vi "INST_PS_SET_CURRENT_LEVEL_4.0.0.vi"(4 "Use OPC(T)":bool, 6 "Instrument Select (Output 1)":string(combo), 7 "SEL_PS":string(combo), 8 "error in (no error)":errorcluster, 9 "Current (0.0)":dbl format="%.2p", 10 "Current (0.0)str":string, 11 "VISA session":refnum<visa-resource-name>) -> (0 "error out":errorcluster, 3 "dup VISA session":refnum<visa-resource-name>)   [LabVIEW 2018]
doc: "This VI configures the DC voltage level the power supply attempts to generate.\n\nVer 3.0.0 supports the E36xx Model and The 6634B based on the GPIB address of idtATE [10-12]"
uses:
  Initialize References/Station References Global.vi
panel:
  out "PSn Model":string
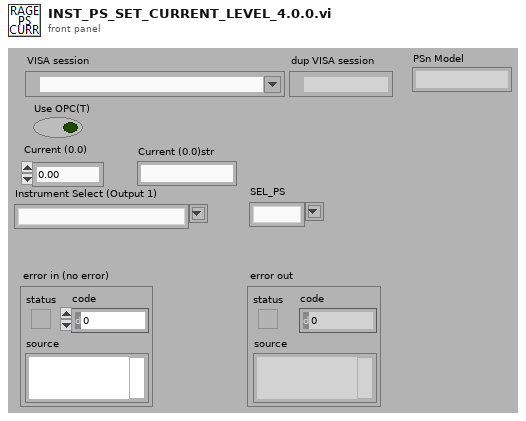
[diagram p1: front panel]
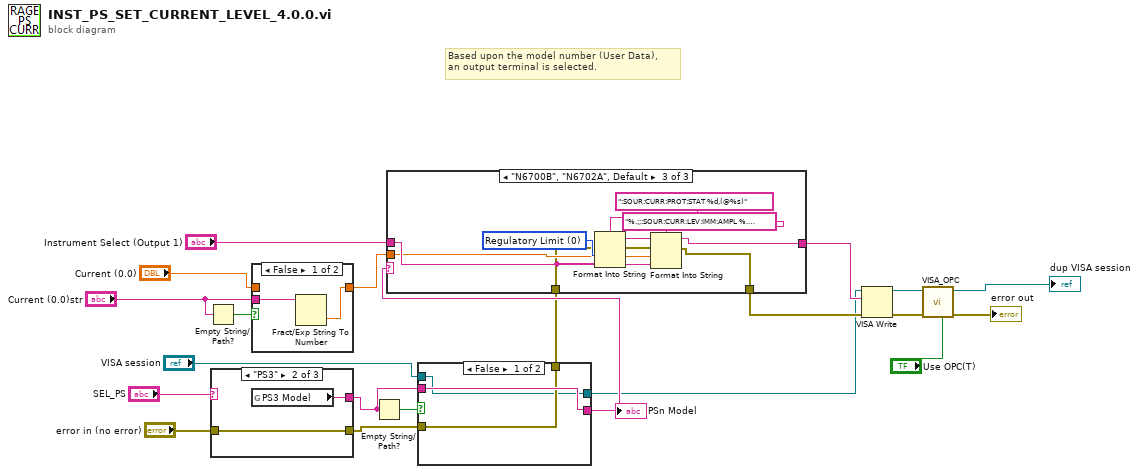
[diagram p0: block diagram]
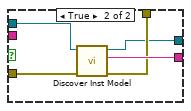
[diagram p2: hidden frame]
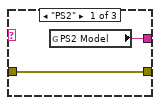
[diagram p3: hidden frame]
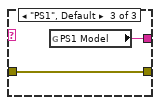
[diagram p4: hidden frame]
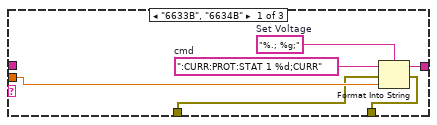
[diagram p5: hidden frame]
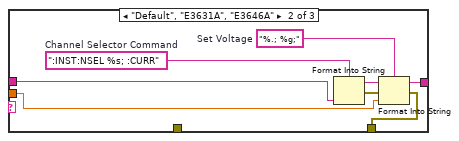
[diagram p6: hidden frame]
diagram:
  # "Based upon the model number (User Data), \nan output terminal is selected."
  n1 = Empty String/Path?(string/path="Current (0.0)str") -> (empty?=w15:bool)
  n2 = case shown="\"PS3\"" "SEL_PS" {
    tunnel: [w23 w25 w27] -> w6
    tunnel: "error in (no error)" -> [w22 w24 w26]
    tunnel: [w22 w24 w26] -> w3
    frame "PS2" {
      n3 = global read "Station References Global.vi" "PS2 Model"() -> (w23:string)
    }
    frame "PS3" {
      n4 = global read "Station References Global.vi" "PS3 Model"() -> (w25:string)
    }
    frame "PS1", Default {
      n5 = global read "Station References Global.vi" "PS1 Model"() -> (w27:string)
    }
  }
  n6 = case shown="False" w15 {
    tunnel: "Current (0.0)str" -> [w29 _]
    tunnel: [w28 w30] -> w14
    tunnel: "Current (0.0)" -> [_ w30]
    frame False {
      n7 = Fract/Exp String To Number(string=w29) -> (number=w28:dbl)  [unwired: 3 in, 1 out]
    }
    frame True {
    }
  }
  n8 = Empty String/Path?(string/path=w6) -> (empty?=w7:bool)
  n9 = case shown="False" w7 {
    tunnel: [w33 w38] -> w5
    tunnel: w6 -> [w33 _]
    tunnel: [w32 w37] -> w4
    tunnel: w3 -> [w32 w36]
    tunnel: "VISA session" -> [w31 w35]
    tunnel: [w31 w34] -> w1
    frame False {
    }
    frame True {
      n10 = call "Discover Inst Model.vi"("error in"=w36, "Session In"=w35) -> ("error out"=w37:errorcluster, "Model #"=w38:string, "Session Out"=w34:refnum<visa-resource-name>)  [unwired: 7 in]
    }
  }
  "PSn Model" <- w5
  n11 = case shown="\"N6700B\", \"N6702A\", Default" w5 {
    tunnel: w14 -> [w41 w49 w57]
    tunnel: "Instrument Select (Output 1)" -> [_ w48 w58]
    tunnel: [w43 w47 w54] -> w12
    tunnel: [w40 w45 w55] -> w9
    tunnel: w4 -> [w39 _ w53]
    frame "6633B", "6634B" {
      w42 = ":CURR:PROT:STAT 1 %d;CURR"  # cmd
      w44 = "%.; %g;"  # Set Voltage
      n12 = Format Into String(format string=w44, initial string=w42, error in=w39, w41) -> (resulting string=w43:string, error out=w40:errorcluster)
    }
    frame "Default", "E3631A", "E3646A" {
      w50 = ":INST:NSEL %s; :CURR"  # Channel Selector Command
      w52 = "%.; %g;"  # Set Voltage
      n13 = Format Into String(format string=w50, w48) -> (resulting string=w51:string, error out=w46:errorcluster)  [unwired: 2 in]
      n14 = Format Into String(format string=w52, initial string=w51, error in=w46, w49) -> (resulting string=w47:string, error out=w45:errorcluster)
    }
    frame "N6700B", "N6702A", Default {
      w60 = 0 items=["Regulatory Limit", "Trip Limit"] ("Behavior (0: Regulatory Limit)")
      n15 = Format Into String(format string=":SOUR:CURR:PROT:STAT %d,(@%s)", error in=w53, w60, w58) -> (resulting string=w62:string, error out=w56:errorcluster)  [unwired: 1 in]
      n16 = Format Into String(format string="%.;;:SOUR:CURR:LEV:IMM:AMPL %.;%Le,(@%s)", initial string=w62, error in=w56, w57, w58) -> (resulting string=w54:string, error out=w55:errorcluster)
    }
  }
  n17 = VISA Write(VISA resource name=w1, write buffer=w12, error in (no error)=w9) -> (VISA resource name out=w21:refnum<visa-resource-name>, error out=w20:errorcluster)  [unwired: 1 out]
  n18 = call "VISA_OPC.vi"("OPC(T)"="Use OPC(T)", "error in"=w20, "Session In"=w21) -> ("error out"=→"error out":errorcluster, "Session Out"=→"dup VISA session":refnum<visa-resource-name>)  [unwired: 6 in, 1 out]
